vi "ManCal.vi"(0 "VISA IN":refnum<visa-resource-name>="GPIB1::16::INSTR", 5 "error in":errorcluster, 7 "Channel":i32=1) -> (14 "VISA Out":refnum<visa-resource-name>="GPIB1::16::INSTR", 19 "error out":errorcluster={"status"=TRUE, "code"=-1073807339, "source"="VISA Read in Check Error.vi->ManCal.vi"})   [LabVIEW 2018, in "PNA-X.lvlib"]
doc: "This VBScript program performs a Guided Calibration using Mechanical standards. While this example is good to use as a starting point for guided mechanical cal, the Guided comprehensive cal example has some advanced features that are not in this program.\n\nThe SCPI commands in this example are sent over a COM interface using the SCPIStringParser object. You do NOT need a GPIB connection to run this example.\n\nThis VBScript (*.vbs) program can be run as a macro in the PNA. To do this, copy the following code into a text editor file such as Notepad and save it on the PNA hard drive as Guided.vbs. Learn how to setup and run the macro.\n\n' Performing a 2-port cal (Ports 1 and 2)\n\nDim app\nDim scpi\n\n' Create / Get the PNA application.\nSet app = CreateObject(\"AgilentPNA835x.Application\")\nSet scpi = app.ScpiStringParser\n\n' Specify the DUT connectors\nscpi.Execute \"sens:corr:coll:guid:conn:port1 \"\"APC 3.5 female\"\" \"\nscpi.Execute \"sens:corr:coll:guid:conn:port2 \"\"APC 3.5 male\"\" \"\n\n' Note: If your PNA has more than 2 ports, you would need to uncomment\n' one or both of these next two lines, to explicitly specify this is\n' just a 2-port cal.\n'scpi.Execute \"sens:corr:coll:guid:conn:port3 \"\"Not used\"\" \"\n'scpi.Execute \"sens:corr:coll:guid:conn:port4 \"\"Not used\"\" \"\nMsgBox \"Connectors defined for Ports 1 and 2\" \n\n' Select the Cal Kit for each port being calibrated.\nscpi.Execute \"sens:corr:coll:guid:ckit:port1 \"\"85052D\"\" \"\nscpi.Execute \"sens:corr:coll:guid:ckit:port2 \"\"85052D\"\" \"\nMsgBox \"Cal kits defined for Ports 1 and 2\"\n\n' Initiate the calibration and query the number of steps\nscpi.Execute \"sens:corr:coll:guid:init\"\nnumSteps = scpi.Execute(\"sens:corr:coll:guid:steps?\")\nMsgBox \"Number of steps is \" + CStr(numSteps)\n\n' Measure the standards\n'The following series of commands shows that standards \n'can be measured in any order. These steps acquire \n'measurement of standards in reverse order.\n'It is easiest to iterate through standards using \n'a For-Next Loop.\nFor i = numSteps To 1\nstep = \"Step \" + CStr(i) + \" of \" + CStr(numSteps)\nstrPrompt = scpi.Execute(\"sens:corr:coll:guid:desc? \" + CStr(i))\nMsgBox strPrompt, vbOKOnly, step\nscpi.Execute \"sens:corr:coll:guid:acq STAN\" + CStr(i)\nNext\n\n' Conclude the calibration\nscpi.Execute \"sens:corr:coll:guid:save\"\nMsgBox \"Cal is done!\""
uses:
  PNA-X.lvlib
  Instance           1 14Saved   ManCal .vi
panel:
  # "Select VNA Visa Addreess"
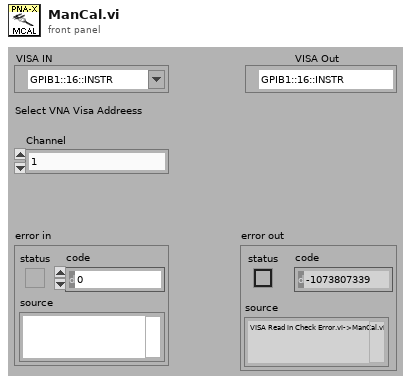
[diagram p1: front panel]
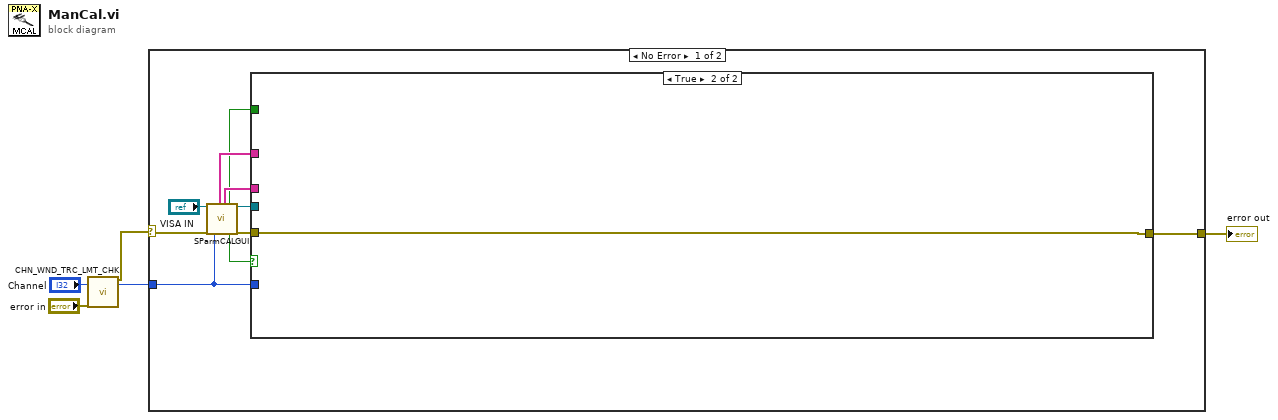
[diagram p0: block diagram]
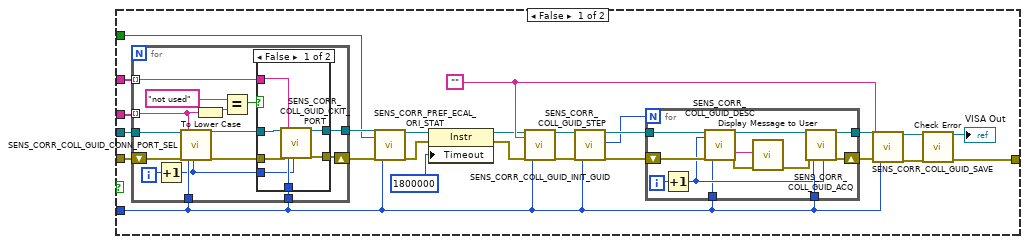
[diagram p2: hidden frame]
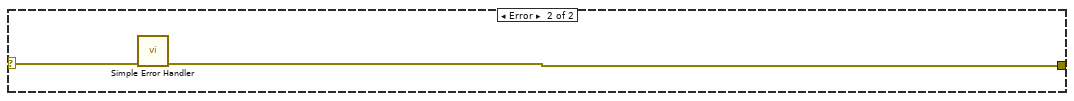
[diagram p4: hidden frame]
diagram:
  n1 = call "CHN_WND_TRC_LMT_CHK.vi"("Channel"="Channel", "error in"="error in") -> ("error out"=w1:errorcluster, "Channel"=w4:i32)  [unwired: 13 in, 3 out]
  n2 = case shown="No Error" w1 {
    selector: w1 -> [w14 w78]
    tunnel: [w15 w79] -> w2
    tunnel: w4 -> [w7 _]
    frame No Error {
      n3 = call "SParmCALGUI.vi"("VNA"="VISA IN", "error in"=w14, "Channel"=w7) -> ("CalKit"=w10:string[], "Conn"=w9:string[], "Orient"=w8:bool, "Exit"=w6:bool, "VNA Out"=w12:refnum<visa-resource-name>, "error out"=w13:errorcluster)  [unwired: 11 in]
      n4 = case shown="True" w6 {
        tunnel: [w30 w77] -> w15
        tunnel: w13 -> [w26 w77]
        tunnel: w12 -> [w25 _]
        tunnel: w10 -> [w24 _]
        tunnel: w9 -> [w23 _]
        tunnel: w8 -> [w22 _]
        tunnel: w7 -> [w16 _]
        frame False {
          w29 = ""
          n5 = for {
            tunnel: w25 -> [w66]
            tunnel: w23 -> [w63] mode=indexing
            shift-right: [w58] -> w27
            shift-left: w26 -> [w67]
            tunnel: w16 -> [w64]
            tunnel: [w56] -> w28
            tunnel: w24 -> [w55] mode=indexing
            tunnel: w16 -> [w54]
            i -> [w65]
            n6 = Increment(x=w65) -> (x+1=w53:i32)
            n7 = call "SENS_CORR_COLL_GUID_CONN_PORT_SEL.vi"("VISA IN"=w66, "error in"=w67, "Port Type"=w63, "Channel"=w64, "Port"=w53) -> ("VISA Out"=w57:refnum<visa-resource-name>, "error out"=w59:errorcluster)  [unwired: 13 in]
            n8 = To Lower Case(string=w63) -> (all lower case string=w62:string)
            n9 = Equal?(x="not used", y=w62) -> (x = y?=w60:bool)
            n10 = case shown="False" w60 {
              tunnel: w59 -> [w74 w75]
              tunnel: [w73 w75] -> w58
              tunnel: w57 -> [w72 w76]
              tunnel: [w71 w76] -> w56
              tunnel: w55 -> [w70 _]
              tunnel: w54 -> [w69 _]
              tunnel: w53 -> [w68 _]
              frame False {
                n11 = call "SENS_CORR_COLL_GUID_CKIT_PORT.vi"("VISA IN"=w72, "error in"=w74, "Ecal ID"=w70, "Channel"=w69, "Port"=w68) -> ("VISA Out"=w71:refnum<visa-resource-name>, "error out"=w73:errorcluster)  [unwired: 13 in]
              }
              frame True {
              }
            }
          }
          n12 = call "SENS_CORR_PREF_ECAL_ORI_STAT.vi"("VISA IN"=w28, "On/Off"=w22, "error in"=w27, "Channel"=w16) -> ("VISA Out"=w21:refnum<visa-resource-name>, "error out"=w18:errorcluster)  [unwired: 14 in]
          n13 = property class="Instr"(reference=w21, error in=w18, "Timeout"=u32 1800000 ("General Settings:Timeout Value")) -> (reference out=w20:refnum<visa-resource-name>, error out=w19:errorcluster)
          n14 = call "SENS_CORR_COLL_GUID_INIT_GUID.vi"("VISA IN"=w20, "Calset"=w29, "error in"=w19, "Channel"=w16) -> ("VISA Out"=w38:refnum<visa-resource-name>, "error out"=w39:errorcluster)  [unwired: 14 in]
          n15 = call "SENS_CORR_COLL_GUID_STEP.vi"("VISA IN"=w38, "error in"=w39, "Channel"=w16) -> ("VISA Out"=w36:refnum<visa-resource-name>, "Data"=w35:i32, "error out"=w37:errorcluster)  [unwired: 14 in]
          n16 = for {
            N: w35 -> [_]
            tunnel: w36 -> [w50]
            tunnel: w16 -> [w51]
            shift-right: [w45] -> w34
            shift-left: w37 -> [w49]
            tunnel: [w44] -> w33
            tunnel: w16 -> [w47]
            i -> [w52]
            n17 = Increment(x=w52) -> (x+1=w48:i32)
            n18 = call "SENS_CORR_COLL_GUID_DESC.vi"("VISA IN"=w50, "Index"=w48, "error in"=w49, "Channel"=w47) -> ("VISA Out"=w46:refnum<visa-resource-name>, "Description"=w41:string, "error out"=w43:errorcluster)  [unwired: 13 in]
            n19 = call "Display Message to User"("error in (no error)"=w43, "Message"=w41) -> ("error out"=w42:errorcluster)  [unwired: 8 in, 1 out]
            n20 = call "SENS_CORR_COLL_GUID_ACQ.vi"("VISA IN"=w46, "error in"=w42, "Channel"=w51, "Standerd"=w48) -> ("VISA Out"=w44:refnum<visa-resource-name>, "error out"=w45:errorcluster)  [unwired: 14 in]
          }
          n21 = call "SENS_CORR_COLL_GUID_SAVE.vi"("VISA IN"=w33, "Calset"=w29, "error in"=w34, "Channel"=w16) -> ("VISA Out"=w31:refnum<visa-resource-name>, "error out"=w32:errorcluster)  [unwired: 14 in]
          n22 = call "Check Error.vi"("VISA Resource Name"=w31, "error in (no error)"=w32) -> ("dup VISA session"=→"VISA Out":refnum<visa-resource-name>, "error out"=w30:errorcluster)  [unwired: 16 in]
        }
        frame True {
        }
      }
    }
    frame Error {
      n23 = call <vilib>:"Simple Error Handler.vi"("error in (no error)"=w78) -> ("error out"=w79:errorcluster)  [unwired: 4 in, 4 out]
    }
  }
  "error out" <- w2
